vi "Write.vi"(8 "error in (no error)":errorcluster, 10 "Write Data":T1, 11 "IP Connection in":refnum<class "IP Connection.lvclass">) -> (0 "error out":errorcluster, 3 "IP Connection out":refnum<class "IP Connection.lvclass">)   [LabVIEW 2011, in "Tinkerforge.lvlib" / "IP Connection.lvclass"]
doc: "This VI writes a message to the TCP/IP connection."
uses:
  IP Connection.lvclass
  Type Definitions/Message.ctl
  IP Connection.lvclass/IP Connection.ctl
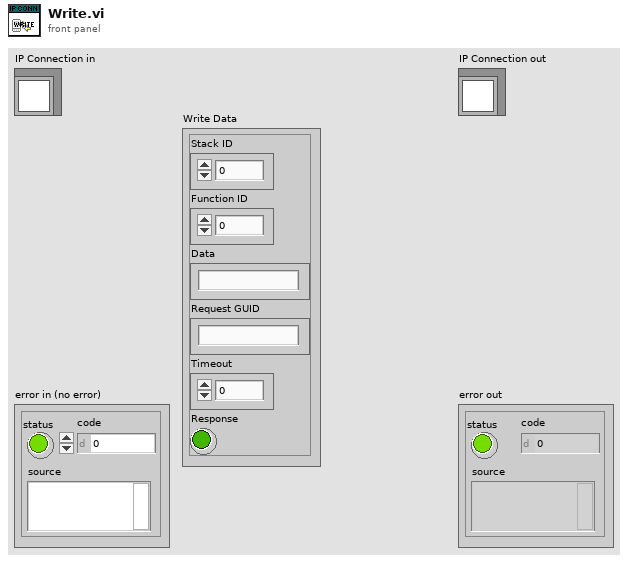
[diagram p1: front panel]
types:
  T1 = typedef "Tinkerforge.lvlib/IP Connection.lvclass/Message.ctl" = cluster{"Stack ID":u8, "Function ID":u8, "Data":string, "Request GUID":string, "Timeout":i32, "Response":bool}
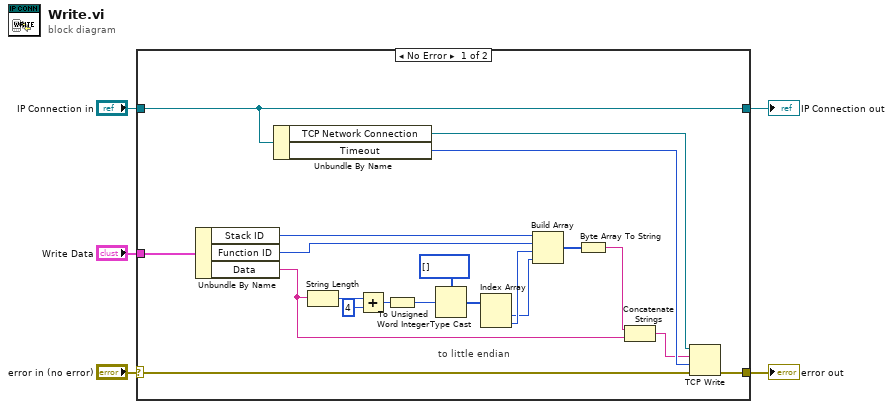
[diagram p0: block diagram]
diagram:
  n1 = case shown="No Error" "error in (no error)" {
    selector: "error in (no error)" -> [w24 w27]
    tunnel: [w23 w27] -> w4
    tunnel: [w25 w26] -> w2
    tunnel: "IP Connection in" -> [w25 w26]
    tunnel: "Write Data" -> [w10 _]
    frame No Error {
      # "to little endian"
      n2 = Unbundle By Name(w10) -> ("Stack ID"=w9:u8, "Function ID"=w8:u8, "Data"=w7:string)
      n3 = Unbundle By Name(w25) -> ("TCP Network Connection"=w22:refnum<k5>, "Timeout"=w21:i32)
      n4 = String Length(string=w7) -> (length=w20:i32)
      n5 = Add(x=w20, y=4) -> (x+y=w18:i32)
      n6 = To Unsigned Word Integer(number=w18) -> (unsigned 16bit integer=w6:u16)
      n7 = Type Cast(type=u8[] [], x=w6) -> (*(type *) &x=w16:u8[])
      n8 = Index Array(array=w16) -> (element #1=w14:u8, element #2=w15:u8)  [unwired: 2 in]
      n9 = Build Array(w9, w8, w15, w14) -> (w13:u8[])
      n10 = Byte Array To String(unsigned byte array=w13) -> (string=w12:string)
      n11 = Concatenate Strings(w12, w7) -> (w11:string)
      n12 = TCP Write(connection ID=w22, data in=w11, error in (no error)=w24, 9:w21) -> (error out=w23:errorcluster)  [unwired: 2 out]
    }
    frame Error {
    }
  }
  "error out" <- w4
  "IP Connection out" <- w2
